vi "oa_FIR Preprocess Filter Kaiser-Bessel Windowed FIR Filter Design.vi"(7 "filter types":T2(ring), 8 "fs [Hz]":dbl=1.0, 10 "ripple specs [dB]":cluster{"pass band":dbl, "stop band":dbl}={"pass band"=0.1, "stop band"=60.0} {"stop band" format="%0.2f"; "pass band" format="%0.2f"}, 11 "freq specs [Hz]":T1={"fpass 1"=0.125, "fstop 1"=0.45, "fpass 2"=0.0, "fstop 2"=0.0} {"fstop 2" format="%0.2f"; "fpass 2" format="%.3f"; "fstop 1" format="%0.2f"; "fpass 1" format="%.3f"}) -> (0 "error":i32, 3 "FIR Windowed Coefficients":dbl[](array[numeric]) format="%0.2f")   [LabVIEW 2017, in "SoundVib_RefDataProcess.lvlib"]
uses:
  <vilib>/addons/Sound and Vibration/Order Analysis/Referece Data Processing/SoundVib_RefDataProcess.lvlib
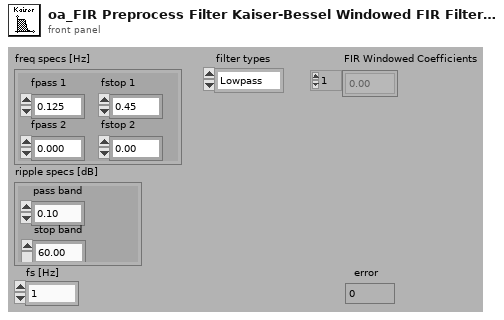
[diagram p1: front panel]
types:
  T1 = cluster{"fpass 1":dbl, "fstop 1":dbl, "fpass 2":dbl, "fstop 2":dbl}
  T2 = enum32{"Lowpass", "Highpass", "Bandpass", "Bandstop"}
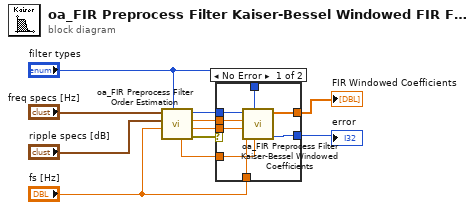
[diagram p0: block diagram]
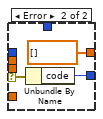
[diagram p2: hidden frame]
diagram:
  n1 = call <vilib>:"oa_FIR Preprocess Filter Order Estimation.vi"("filter types"="filter types", "fs [Hz]"="fs [Hz]", "ripple specs [dB]"="ripple specs [dB]", "freq specs [Hz]"="freq specs [Hz]") -> ("error out"=w1:errorcluster, "low cutoff freq: fl"=w9:dbl, "high cutoff freq: fh"=w10:dbl, "estimated order"=w11:i32, "beta"=w8:dbl)  [unwired: 3 in]
  n2 = case shown="No Error" w1 {
    selector: w1 -> [_ w21]
    tunnel: w11 -> [w19 _]
    tunnel: w10 -> [w18 _]
    tunnel: w9 -> [w17 _]
    tunnel: w8 -> [w16 _]
    tunnel: [w15 dbl[] [] ("FIR Windowed Coefficients")] -> w5
    tunnel: [w14 w20] -> w4
    tunnel: "filter types" -> [w13 _]
    tunnel: "fs [Hz]" -> [w12 _]
    frame No Error {
      n3 = call <vilib>:"oa_FIR Preprocess Filter Kaiser-Bessel Windowed Coefficients.vi"("beta"=w16, "filter type"=w13, "sampling freq: fs"=w12, "low cutoff freq: fl"=w17, "high cutoff freq: fh"=w18, "order"=w19) -> ("error"=w14:i32, "FIR Windowed Coefficients"=w15:dbl[])  [unwired: 4 in]
    }
    frame Error {
      n4 = Unbundle By Name(w21) -> ("code"=w20:i32)
    }
  }
  "FIR Windowed Coefficients" <- w5
  "error" <- w4
